vi "ADIS16448 Compute Calibration Offsetsvi.vi"(11 "Array":T2(array[cluster])) -> (2 "Variance":T1, 3 "DC value":cluster{"mean":dbl, "mean":dbl, "mean":dbl})   [LabVIEW 2019]
uses:
  <vilib>/Analysis/NI_AALBase.lvlib
panel:
  in  "skip index":i32=3
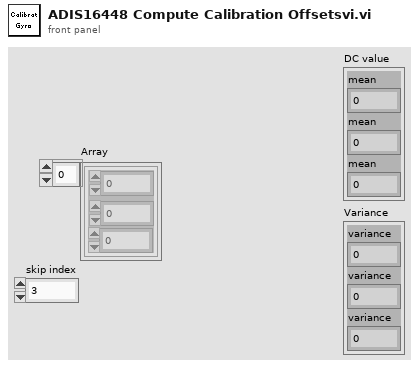
[diagram p1: front panel]
types:
  T1 = cluster{"variance":dbl, "variance":dbl, "variance":dbl}
  T2 = cluster{"Numeric":dbl, "Numeric 2":dbl, "Numeric 3":dbl}[]
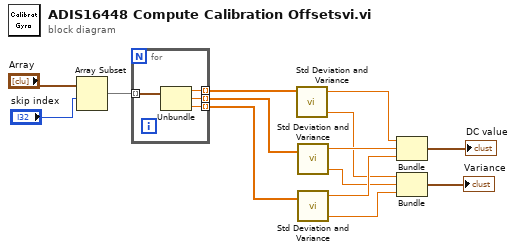
[diagram p0: block diagram]
diagram:
  n1 = Array Subset(array="Array", index="skip index") -> (w12:T2)  [unwired: 1 in]
  n2 = for {
    tunnel: w12 -> [w18] mode=indexing
    tunnel: [w17] -> w11 mode=indexing
    tunnel: [w16] -> w10 mode=indexing
    tunnel: [w15] -> w9 mode=indexing
    n3 = Unbundle(w18) -> ("Numeric"=w17:dbl, "Numeric 2"=w16:dbl, "Numeric 3"=w15:dbl)
  }
  n4 = call <vilib>:"Std Deviation and Variance.vi"("X"=w11) -> ("mean"=w8:dbl, "variance"=w5:dbl)  [unwired: 1 in, 1 out]
  n5 = call <vilib>:"Std Deviation and Variance.vi"("X"=w10) -> ("mean"=w7:dbl, "variance"=w4:dbl)  [unwired: 1 in, 1 out]
  n6 = call <vilib>:"Std Deviation and Variance.vi"("X"=w9) -> ("mean"=w6:dbl, "variance"=w3:dbl)  [unwired: 1 in, 1 out]
  n7 = Bundle("mean"=w8, "mean"=w7, "mean"=w6) -> (→"DC value":cluster{"mean":dbl, "mean":dbl, "mean":dbl})  [unwired: 1 in]
  n8 = Bundle("variance"=w5, "variance"=w4, "variance"=w3) -> (→"Variance":T1)  [unwired: 1 in]
